vi "processSubDataPublish.vi"(8 "error in (no error)":errorcluster, 11 "MiddlewareSVThisComponent in":refnum<class "MiddlewareSVThisComponent.lvclass">) -> (0 "error out":errorcluster, 3 "MiddlewareSVThisComponent out":refnum<class "MiddlewareSVThisComponent.lvclass">)   [LabVIEW 2015, in "MiddlewareSVThisComponent.lvclass"]
uses:
  MiddlewareSVThisComponent.lvclass
  ComponentTemplateCore/ComponentModel/ComponentModel/Middleware/Middleware.lvclass/Middleware.ctl
  ComponentTemplateCore/ComponentModel/ComponentModel/MiddlewareProcessEvent/MiddlewareProcessEvent.lvclass/MiddlewareProcessEvent.ctl
  MiddlewareSVThisComponent.lvclass/MiddlewareSVThisComponent.ctl
  PubSubDataEvent/PubSubDataEvent.lvclass/PubSubDataEvent.ctl
  <vilib>/Utility/error.llb/DialogType.ctl
  Typedefs/SubDataSV.ctl
  ComponentTemplateCore/ComponentModel/ComponentModel/Middleware/Middleware.lvclass
  ComponentTemplateCore/ComponentModel/ComponentModel/MiddlewareProcessEvent/MiddlewareProcessEvent.lvclass
  PubSubDataEvent/PubSubDataEvent.lvclass
  Typedefs/EXATypedefs.lvlib
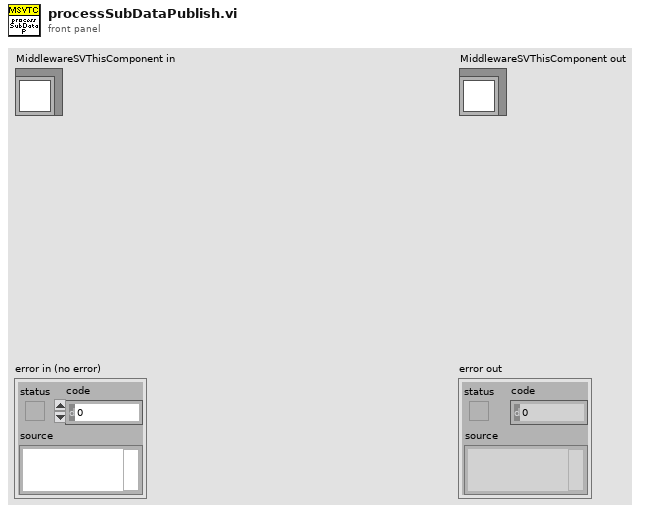
[diagram p1: front panel]
types:
  T1 = typedef "EXATypedefs.lvlib/SubDataEvents.ctl" = cluster{"ClearError":refnum<user-event>, "Disable":refnum<user-event>, "Enable":refnum<user-event>, "Exit":refnum<user-event>, "GoToStandby":refnum<user-event>, "HeartbeatIn":refnum<user-event>, "Start":refnum<user-event>}
  T2 = typedef "MiddlewareProcessEvents.ctl" = cluster{"disconnect":refnum<user-event>, "error":refnum<user-event>}
  T3 = typedef "EXATypedefs.lvlib/SubDataSV.ctl" = enum16{"ClearError", "Disable", "Enable", "Exit", "GoToStandby", "HeartbeatIn", "Start"}
  T4 = typedef "DialogType.ctl" = u16
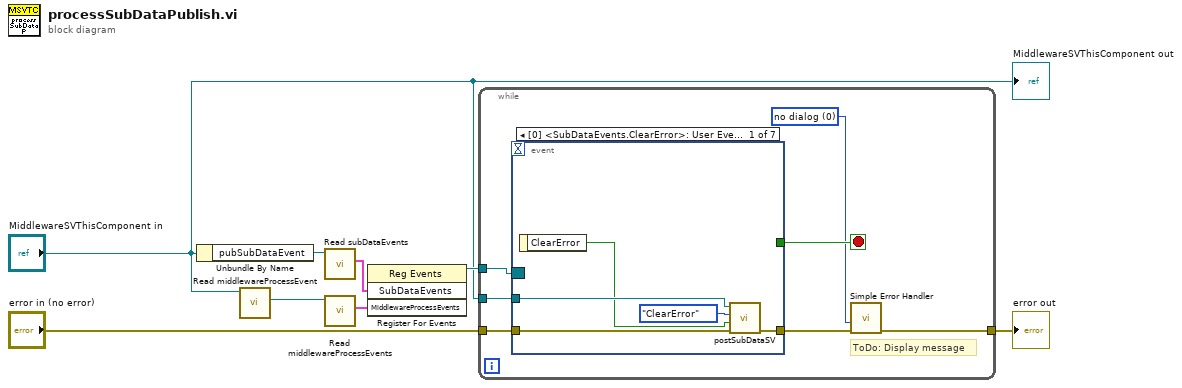
[diagram p0: block diagram]
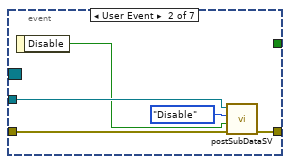
[diagram p2: hidden frame]
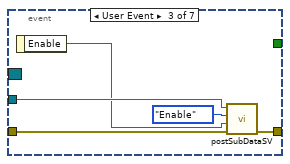
[diagram p3: hidden frame]
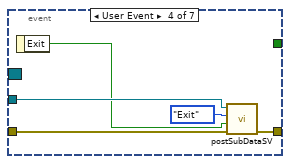
[diagram p4: hidden frame]
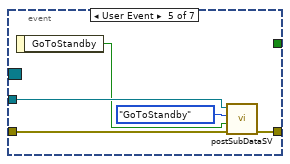
[diagram p5: hidden frame]
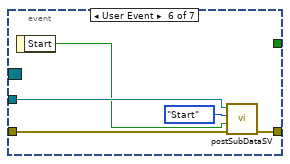
[diagram p6: hidden frame]
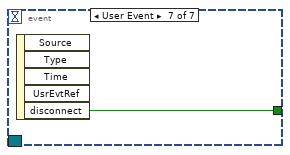
[diagram p7: hidden frame]
diagram:
  n1 = Unbundle By Name("MiddlewareSVThisComponent in") -> ("pubSubDataEvent"=w3:refnum<class "PubSubDataEvent.lvclass">)
  n2 = call "Read middlewareProcessEvent.vi"("Middleware in"="MiddlewareSVThisComponent in") -> ("middlewareProcessEvent"=w6:refnum<class "MiddlewareProcessEvent.lvclass">)  [unwired: 9 in, 1 out]
  n3 = call "Read subDataEvents.vi"("PubSubDataEvent in"=w3) -> ("SubDataEvents"=w2:T1)  [unwired: 9 in, 1 out]
  n4 = call "Read middlewareProcessEvents.vi"("MiddlewareProcessEvent in"=w6) -> ("MiddlewareProcessEvents"=w5:T2)  [unwired: 9 in, 1 out]
  n5 = register-events(w2, w5) -> (reference out=w8:refnum<event-registration>)  [unwired: 2 in, 1 out]
  n6 = while {
    tunnel: w8 -> [w15]
    tunnel: "error in (no error)" -> [w12]
    tunnel: "MiddlewareSVThisComponent in" -> [w10]
    tunnel: [w9] -> w1
    stop <- w14 stop-if-true
    w13 = T4 0 items=["no dialog", "OK message", "continue or stop message", "OK message + warnings", "continue/stop + warnings"] ("type of dialog (OK msg:1)")
    # "ToDo: Display message"
    n7 = event shown="[0] <SubDataEvents.ClearError>: User Event" {
      selector: w15 -> [_ _ _ _ _ _ _]
      dyn-events: _ -> [_ _ _ _ _ _ _]
      timeout: _ -> [_ _ _ _ _ _ _]
      tunnel: [_ _ _ _ _ _ w46] -> w14
      tunnel: w12 -> [w19 w24 w29 w34 w39 w44 _]
      tunnel: [w18 w23 w28 w33 w38 w43 _] -> w11
      tunnel: w10 -> [w20 w25 w30 w35 w40 w45 _]
      event User Event {
        n8 = event-data() -> ("ClearError"=w17:bool)  [unwired: 1 in]
        n9 = call "postSubDataSV.vi"("error in (no error)"=w19, "value"=w17, "subDataSV"=SubDataSV."ClearError" ("SubDataSV"), "MiddlewareSVThisComponent in"=w20) -> ("error out"=w18:errorcluster)  [unwired: 6 in, 1 out]
      }
      event User Event {
        n10 = event-data() -> ("Disable"=w22:bool)  [unwired: 1 in]
        n11 = call "postSubDataSV.vi"("error in (no error)"=w24, "value"=w22, "subDataSV"=SubDataSV."Disable" ("SubDataSV"), "MiddlewareSVThisComponent in"=w25) -> ("error out"=w23:errorcluster)  [unwired: 6 in, 1 out]
      }
      event User Event {
        n12 = event-data() -> ("Enable"=w27:bool)  [unwired: 1 in]
        n13 = call "postSubDataSV.vi"("error in (no error)"=w29, "value"=w27, "subDataSV"=SubDataSV."Enable" ("SubDataSV"), "MiddlewareSVThisComponent in"=w30) -> ("error out"=w28:errorcluster)  [unwired: 6 in, 1 out]
      }
      event User Event {
        n14 = event-data() -> ("Exit"=w32:bool)  [unwired: 1 in]
        n15 = call "postSubDataSV.vi"("error in (no error)"=w34, "value"=w32, "subDataSV"=SubDataSV."Exit" ("SubDataSV"), "MiddlewareSVThisComponent in"=w35) -> ("error out"=w33:errorcluster)  [unwired: 6 in, 1 out]
      }
      event User Event {
        n16 = event-data() -> ("GoToStandby"=w37:bool)  [unwired: 1 in]
        n17 = call "postSubDataSV.vi"("error in (no error)"=w39, "value"=w37, "subDataSV"=SubDataSV."GoToStandby" ("SubDataSV"), "MiddlewareSVThisComponent in"=w40) -> ("error out"=w38:errorcluster)  [unwired: 6 in, 1 out]
      }
      event User Event {
        n18 = event-data() -> ("Start"=w42:bool)  [unwired: 1 in]
        n19 = call "postSubDataSV.vi"("error in (no error)"=w44, "value"=w42, "subDataSV"=SubDataSV."Start" ("SubDataSV"), "MiddlewareSVThisComponent in"=w45) -> ("error out"=w43:errorcluster)  [unwired: 6 in, 1 out]
      }
      event User Event {
        n20 = event-data() -> ("disconnect"=w46:bool)  [unwired: 1 in, 4 out]
      }
    }
    n21 = call <vilib>:"Simple Error Handler.vi"("type of dialog (OK msg:1)"=w13, "error in (no error)"=w11) -> ("error out"=w9:errorcluster)  [unwired: 3 in, 4 out]
  }
  "error out" <- w1
  "MiddlewareSVThisComponent out" <- "MiddlewareSVThisComponent in"
